vi "SMU.GetCurrent.vi"(8 "error in (no error)":errorcluster, 11 "SMU.Simulated in":refnum<class "SMU.Simulated.lvclass">) -> (0 "error out":errorcluster, 2 "Current, A":dbl format="%#_13g", 3 "SMU.Simulated out":refnum<class "SMU.Simulated.lvclass">)   [LabVIEW 2017, in "SMU.Simulated.lvclass"]
uses:
  SMU.Simulated.lvclass
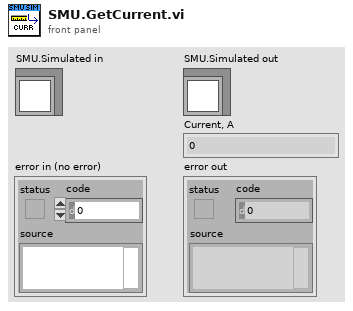
[diagram p1: front panel]
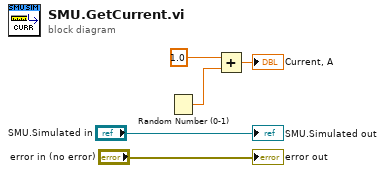
[diagram p0: block diagram]
diagram:
  n1 = Random Number (0-1)() -> (number: 0 to 1=w3:dbl)
  n2 = Add(x=1.0, y=w3) -> (x+y=→"Current, A":dbl)
  "error out" <- "error in (no error)"
  "SMU.Simulated out" <- "SMU.Simulated in"
